vi "Abort Cal Point.vi"(0 "CART TCP Connection In":refnum<k5>, 11 "error in (no error)":errorcluster) -> (4 "CART TCP Connection Out":refnum<k5>, 8 "TCP Messages":string[](array[string]), 15 "error out":errorcluster)   [LabVIEW 2011]
uses:
  Controls/NART Response Subtype.ctl
  Controls/NART TCP Response Types.ctl
  CART/Controls/Parameter.ctl
  SubVIs/NART Constants.vi
  ART2 Test Panel.lvlib
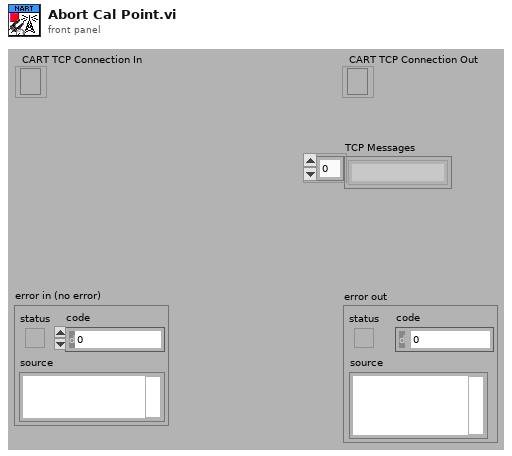
[diagram p1: front panel]
types:
  T1 = typedef "ART2 Test Panel.lvlib/NART Response Subtype.ctl" = enum16{"NONE", "OK", "ON", "OFF", "BEGIN", "DONE"}
  T2 = typedef "ART2 Test Panel.lvlib/NART TCP Response Types.ctl" = enum16{"DEBUG", "CONTROL", "INFO", "WARNING", "ERROR", "NONE"}
  T3 = typedef "ART2 Test Panel.lvlib/Parameter.ctl" = cluster{"Name":string, "Type":enum16{"decimal", "string", "float", "hex"}}
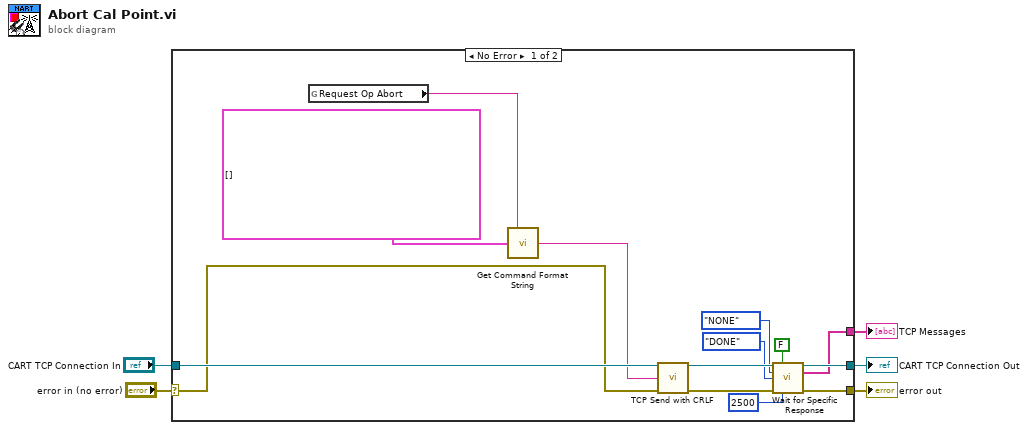
[diagram p0: block diagram]
diagram:
  n1 = case shown="No Error" "error in (no error)" {
    selector: "error in (no error)" -> [w16 w21]
    tunnel: [w13 w21] -> w4
    tunnel: "CART TCP Connection In" -> [w19 w20]
    tunnel: [w14 w20] -> w2
    tunnel: [w9 _] -> w1
    frame No Error {
      n2 = global read "NART Constants.vi" "Request Op Abort"() -> (w6:string)
      n3 = call "Get Command Format String.vi"("Command"=w6, "Parameters"=T3[] []) -> ("Command Format String"=w17:string)  [unwired: 13 in]
      n4 = call "TCP Send with CRLF.vi"("CART TCP Connection"=w19, "data in"=w17, "error IO"=w16) -> ("CART TCP Connection Out"=w15:refnum<k5>, "error out"=w12:errorcluster)  [unwired: 11 in]
      n5 = call "Wait for Specific Response.vi"("TCP Connection In"=w15, "Next response (t)"=FALSE, "Expected Type"=NART_TCP_Response_Types."NONE" ("Expected Response"), "Expected Subtype (none)"=NART_Response_Subtype."DONE" ("Response Subtype"), "error in"=w12, "Timeout (250 ms)"=2500) -> ("TCP Connection Out"=w14:refnum<k5>, "TCP Messages"=w9:string[], "error out"=w13:errorcluster)  [unwired: 6 in, 1 out]
    }
    frame Error {
    }
  }
  "error out" <- w4
  "CART TCP Connection Out" <- w2
  "TCP Messages" <- w1
